vi "Read_Current_Arm_Position.vi"(10 "error in (no error)":errorcluster, 11 "Machine In":refnum<visa-resource-name>) -> (1 "read buffer":string, 2 "error out":errorcluster, 3 "Machine Out":refnum<visa-resource-name>)   [LabVIEW 2018]
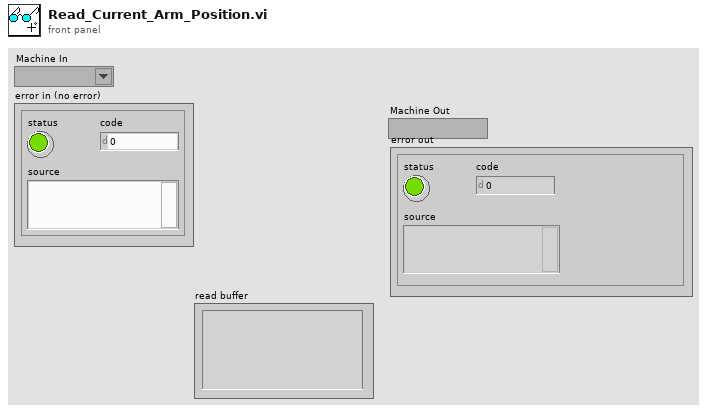
[diagram p1: front panel]
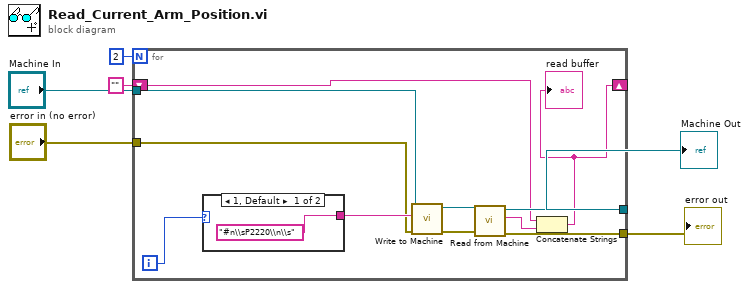
[diagram p0: block diagram]
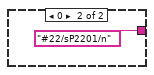
[diagram p2: hidden frame]
diagram:
  n1 = for {
    N: 2 -> [_]
    tunnel: [w14] -> w6
    tunnel: [w13] -> w5
    tunnel: "error in (no error)" -> [w12]
    tunnel: "Machine In" -> [w11]
    shift-right: [w7] -> _
    shift-left: "" ("read buffer") -> [w8]
    i -> [w10]
    n2 = case shown="1, Default" w10 {
      tunnel: ["#n\\sP2220\\n\\s" ("G-Code String In") "#22/sP2201/n" ("G-Code String In")] -> w17
      frame 1, Default {
      }
      frame 0 {
      }
    }
    n3 = call "Write to Machine .vi"("error in (no error)"=w12, "G-Code String In"=w17, "Machine In"=w11) -> ("error out"=w15:errorcluster, "Machine Out"=w16:refnum<visa-resource-name>)  [unwired: 7 in]
    n4 = call "Read from Machine.vi"("error in (no error)"=w15, "Machine In"=w16) -> ("error out"=w13:errorcluster, "read buffer"=w9:string, "Machine Out"=w14:refnum<visa-resource-name>)  [unwired: 7 in]
    n5 = Concatenate Strings(w8, w9) -> (w7:string)
    "read buffer" <- w7
  }
  "Machine Out" <- w6
  "error out" <- w5
